vi "Find Result File Name.vi"(8 "Error In":errorcluster, 9 "Extension":string, 10 "Prefix":string="US", 11 "Directory":path) -> (0 "error out":errorcluster, 1 "File No.":i32, 2 "File Name":string, 3 "Result File Path":path)   [LabVIEW 2016]
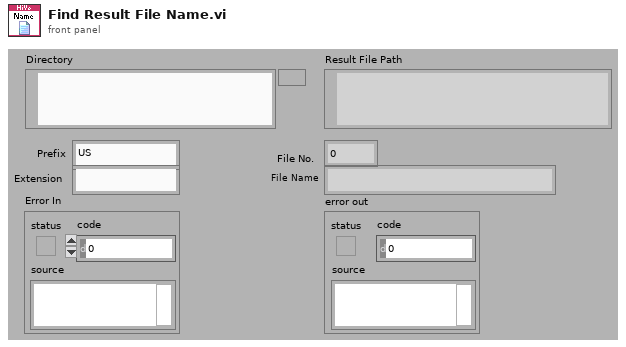
[diagram p1: front panel]
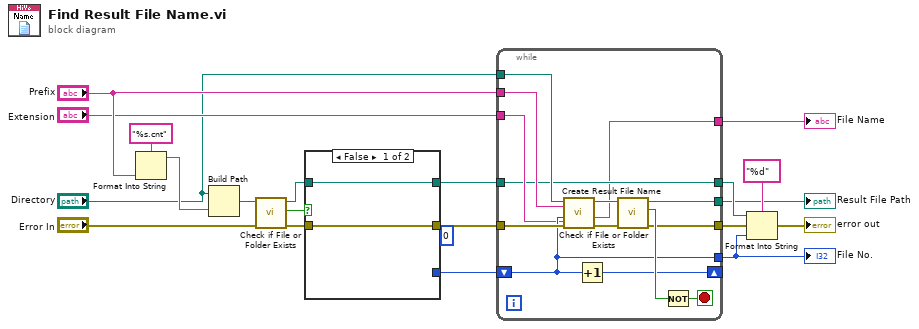
[diagram p0: block diagram]
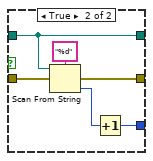
[diagram p2: hidden frame]
diagram:
  n1 = Format Into String(format string="%s.cnt", "Prefix") -> (resulting string=w19:string)  [unwired: 2 in, 1 out]
  n2 = Build Path(base path="Directory", name or relative path=w19) -> (appended path=w17:path)
  n3 = call <vilib>:"Check if File or Folder Exists.vi"("error in (no error)"="Error In", "path"=w17) -> ("error out"=w16:errorcluster, "file or folder exists?"=w18:bool, "dup path"=w15:path)  [unwired: 7 in]
  n4 = case shown="False" w18 {
    tunnel: [w23 w28] -> w8
    tunnel: w16 -> [w23 w27]
    tunnel: w15 -> [w21 w25]
    tunnel: [0 w26] -> w13
    tunnel: [w21 w25] -> w6
    frame False {
    }
    frame True {
      n5 = Scan From String("%d" ("Format String"), w25, w27) -> (w28:errorcluster, output 1=w24:i32)  [unwired: 1 in, 1 out]
      n6 = Increment(x=w24) -> (x+1=w26:i32)
    }
  }
  n7 = while {
    tunnel: w8 -> [w43]
    tunnel: "Directory" -> [w42]
    tunnel: "Prefix" -> [w41]
    tunnel: [w36] -> w4
    shift-right: [w35] -> _
    shift-left: w13 -> [w33]
    tunnel: [w34] -> w10
    tunnel: [w33] -> w11
    tunnel: "Extension" -> [w32]
    tunnel: w6 -> [w31]
    tunnel: [w31] -> w5
    tunnel: [w30] -> w3
    stop <- w37 stop-if-true
    n8 = call "Create Result File Name.vi"("Extension"=w32, "error in (no error)"=w43, "File No."=w33, "Prefix"=w41, "Result Directory"=w42) -> ("error out"=w40:errorcluster, "File Name"=w30:string, "Result File Path"=w39:path)  [unwired: 4 in]
    n9 = Increment(x=w33) -> (x+1=w35:i32)
    n10 = call <vilib>:"Check if File or Folder Exists.vi"("error in (no error)"=w40, "path"=w39) -> ("error out"=w34:errorcluster, "file or folder exists?"=w38:bool, "dup path"=w36:path)  [unwired: 7 in]
    n11 = Not(x=w38) -> (.not. x?=w37:bool)
  }
  "File No." <- w11
  "Result File Path" <- w4
  "File Name" <- w3
  n12 = Format Into String(format string="%d" ("Format String"), initial string=w5, error in=w10, w11) -> (error out=→"error out":errorcluster)  [unwired: 1 out]
